vi "average_with_corrections_expSD.vi"(8 "error in (no error)":errorcluster, 10 "sigma":dbl, 11 "all exp to average":refnum<class "Experiment.lvclass">[](array[class])) -> (0 "sortie d'erreur":errorcluster, 2 "timedelays longest":dbl[](array[numeric]), 3 "averaged without bad points":dbl[][](array[numeric]))   [LabVIEW 2020]
uses:
  Classes/Experiments/Experiment.lvclass
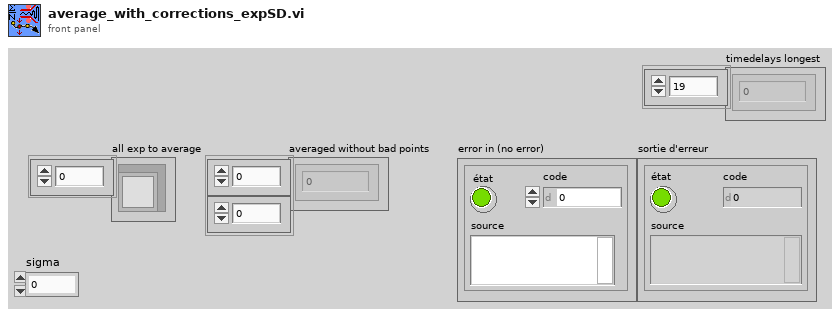
[diagram p1: front panel]
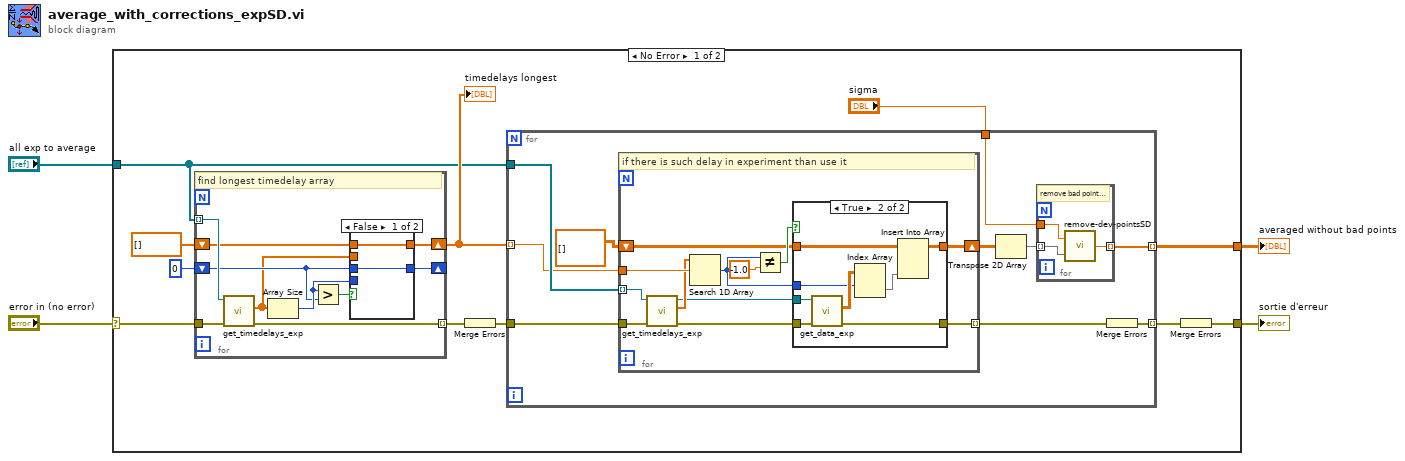
[diagram p0: block diagram]
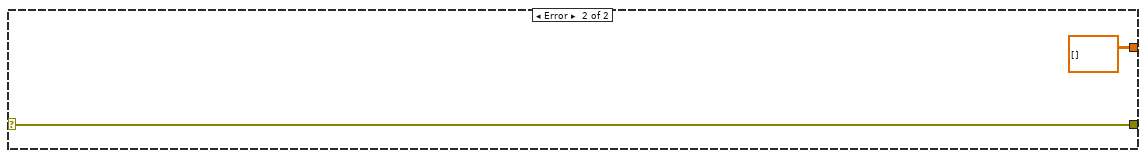
[diagram p4: hidden frame]
diagram:
  n1 = case shown="No Error" "error in (no error)" {
    selector: "error in (no error)" -> [w6 w66]
    tunnel: "all exp to average" -> [w12 _]
    tunnel: [w11 dbl[][] []] -> w3
    tunnel: [w9 w66] -> w2
    frame No Error {
      n2 = for {
        tunnel: w12 -> [w60] mode=indexing
        shift-right: [w58] -> _
        shift-left: 0 -> [w56]
        shift-right: [w54] -> w13
        shift-left: dbl[] [] ("timedelays") -> [w53]
        tunnel: w6 -> [w52]
        tunnel: [w51] -> w8 mode=indexing
        # "find longest timedelay array"
        n3 = call "get_timedelays_exp.vi"("error in (no error)"=w52, "Experiment.lvclass in"=w60) -> ("error out"=w51:errorcluster, "timedelays"=w55:dbl[])  [unwired: 7 in, 1 out]
        n4 = Array Size(array=w55) -> (size(s)=w57:i32)
        n5 = Greater?(x=w57, y=w56) -> (0:w59:bool)
        n6 = case shown="False" w59 {
          tunnel: [w62 w64] -> w58
          tunnel: w57 -> [_ w64]
          tunnel: w56 -> [w62 _]
          tunnel: w55 -> [_ w63]
          tunnel: [w61 w63] -> w54
          tunnel: w53 -> [w61 _]
          frame False {
          }
          frame True {
          }
        }
      }
      "timedelays longest" <- w13
      n7 = Merge Errors(w8) -> (w7:errorcluster)
      n8 = for {
        tunnel: w13 -> [w24] mode=indexing
        tunnel: w12 -> [w25]
        tunnel: [w20] -> w11 mode=indexing
        tunnel: [w18] -> w10 mode=indexing
        tunnel: w7 -> [w17]
        tunnel: "sigma" -> [w16]
        n9 = for {
          tunnel: w25 -> [w36] mode=indexing
          tunnel: w24 -> [w40]
          shift-right: [w32] -> w22
          shift-left: dbl[][] [] ("Data") -> [w33]
          tunnel: w17 -> [w31]
          tunnel: [w30] -> w19 mode=indexing
          # "if there is such delay in experiment than use it"
          n10 = call "get_timedelays_exp.vi"("error in (no error)"=w31, "Experiment.lvclass in"=w36) -> ("error out"=w35:errorcluster, "timedelays"=w39:dbl[], "Experiment.lvclass out"=w29:refnum<class "Experiment.lvclass">)  [unwired: 7 in]
          n11 = Search 1D Array(1D array=w39, element=w40) -> (index of element=w34:i32)  [unwired: 1 in]
          n12 = Not Equal?(x=w34, y=-1.0) -> (x != y?=w37:bool)
          n13 = case shown="True" w37 {
            tunnel: w29 -> [_ w50]
            tunnel: w35 -> [w41 w49]
            tunnel: w34 -> [_ w47]
            tunnel: w33 -> [w42 w45]
            tunnel: [w42 w44] -> w32
            tunnel: [w41 w43] -> w30
            frame False {
            }
            frame True {
              n14 = call "get_data_exp.vi"("error in (no error)"=w49, "Experiment.lvclass in"=w50) -> ("error out"=w43:errorcluster, "Data"=w48:sgl[][])  [unwired: 7 in, 1 out]
              n15 = Index Array(array=w48, index (row)=w47) -> (element=w46:sgl[])  [unwired: 1 in]
              n16 = Insert Into Array(array=w45, new element=w46) -> (w44:dbl[][])  [unwired: 2 in]
            }
          }
        }
        n17 = Transpose 2D Array(2D array=w22) -> (transposed array=w21:dbl[][])
        n18 = for {
          tunnel: w21 -> [w28] mode=indexing
          tunnel: [w27] -> w20 mode=indexing
          tunnel: w16 -> [w26]
          # "remove bad points and average"
          n19 = call "remove-dev-pointsSD.vi"("IN data lamda at ceratin time"=w28, "sigma"=w26) -> ("Average without bad points"=w27:dbl)
        }
        n20 = Merge Errors(w19) -> (w18:errorcluster)
      }
      n21 = Merge Errors(w10) -> (w9:errorcluster)
    }
    frame Error {
    }
  }
  "averaged without bad points" <- w3
  "sortie d'erreur" <- w2
